vi "MFRDA Mass Flow Rate of Dry Air in Humid Air (Kg to S).vi"(1 "Gas Presure":dbl[unit]=80000.0 min=80000.0 max=120000.0, 2 "Tceg":dbl[unit], 3 "MFRHA\nMass Flow Rate of Humid Air (Kg/s)":dbl[unit], 4 "RH":dbl) -> (0 "MFRDA":dbl[unit])   [LabVIEW 2018]
panel:
  out "MFRDA\nMass Flow Rate of Dry Air in Humid Air\nMFRDA=MFRHA/(1+HR);":dbl[unit](knob) scale=0.0..10.0
  out "Temprature Of Input Air\nKelvin Degree":dbl[unit](slide) scale=273.0..373.0
  out "Tk":dbl[unit]
  out "Temprature Of Input Air\nCentigrade Degree":dbl[unit](slide) scale=0.0..100.0
  out "Humidity of Input Air":dbl(knob) scale=0.0..100.0
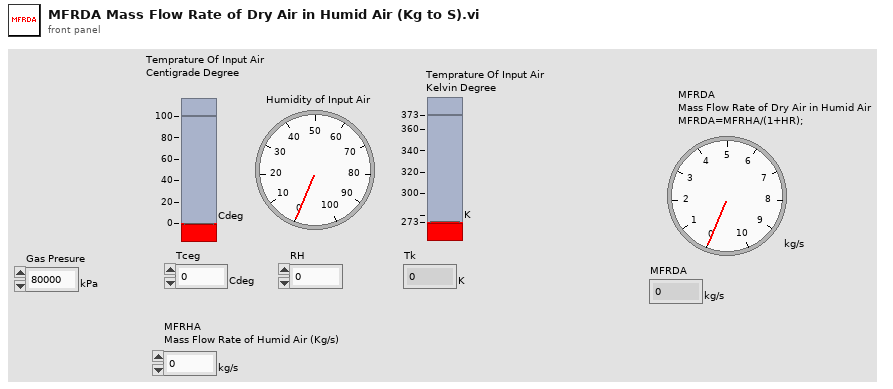
[diagram p1: front panel]
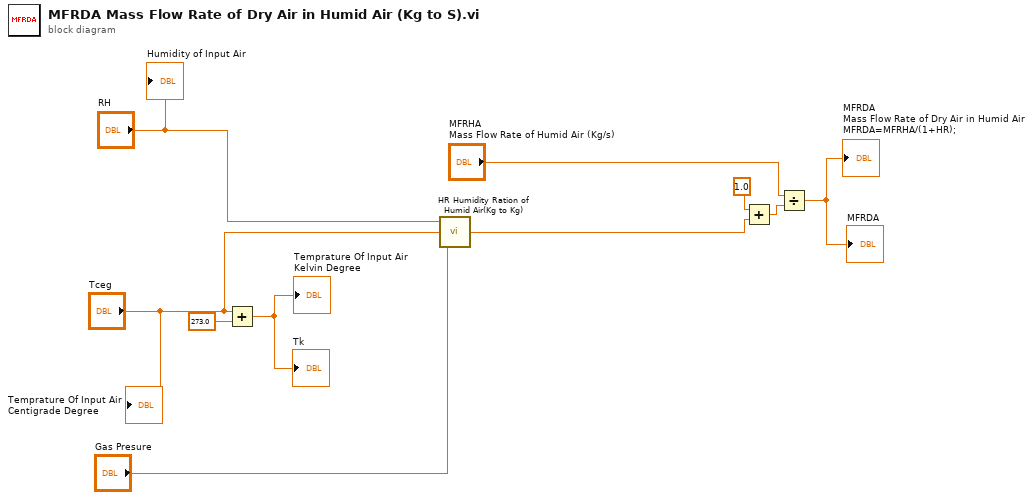
[diagram p0: block diagram]
diagram:
  n1 = Add(x="Tceg", y=dbl[unit] 273.0) -> (x+y=→"Tk" →"Temprature Of Input Air\nKelvin Degree":dbl[unit])
  n2 = call "HR Humidity Ration of Humid Air(Kg to Kg).vi"("Gas Presure"="Gas Presure", "Tceg"="Tceg", "RH"="RH") -> ("HR"=w4:dbl)
  n3 = Add(x=1.0, y=w4) -> (x+y=w8:dbl)
  n4 = Divide(x="MFRHA\nMass Flow Rate of Humid Air (Kg/s)", y=w8) -> (x/y=→"MFRDA\nMass Flow Rate of Dry Air in Humid Air\nMFRDA=MFRHA/(1+HR);" →"MFRDA":dbl[unit])
  "Humidity of Input Air" <- "RH"
  "Temprature Of Input Air\nCentigrade Degree" <- "Tceg"
